vi "start.vi"(8 "error in (no error)":errorcluster, 11 "NetworkProEm in":refnum<class "Network_ProEm_WinX32.lvclass">) -> (0 "error out":errorcluster, 3 "NetworkProEM out":refnum<class "Network_ProEm_WinX32.lvclass">)   [LabVIEW 2009, in "Hardware.lvlib" / "HWControllers.lvlib" / "Network_ProEm_WinX32.lvclass"]
uses:
  Network_ProEm_WinX32.lvclass
  Channels/Camera/Camera/Camera.lvclass
  NetworkCamera.lvclass
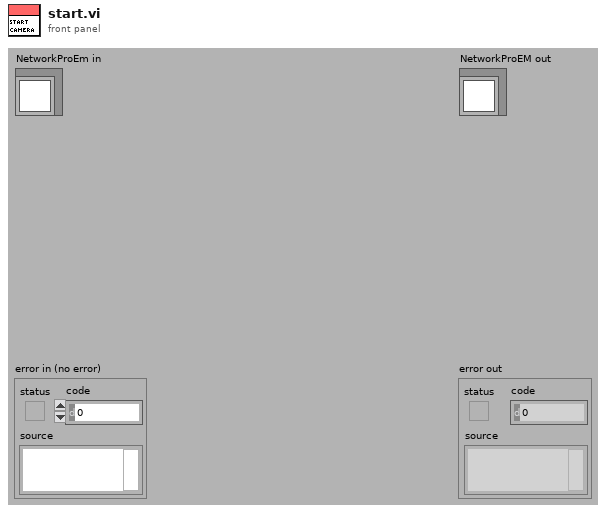
[diagram p1: front panel]
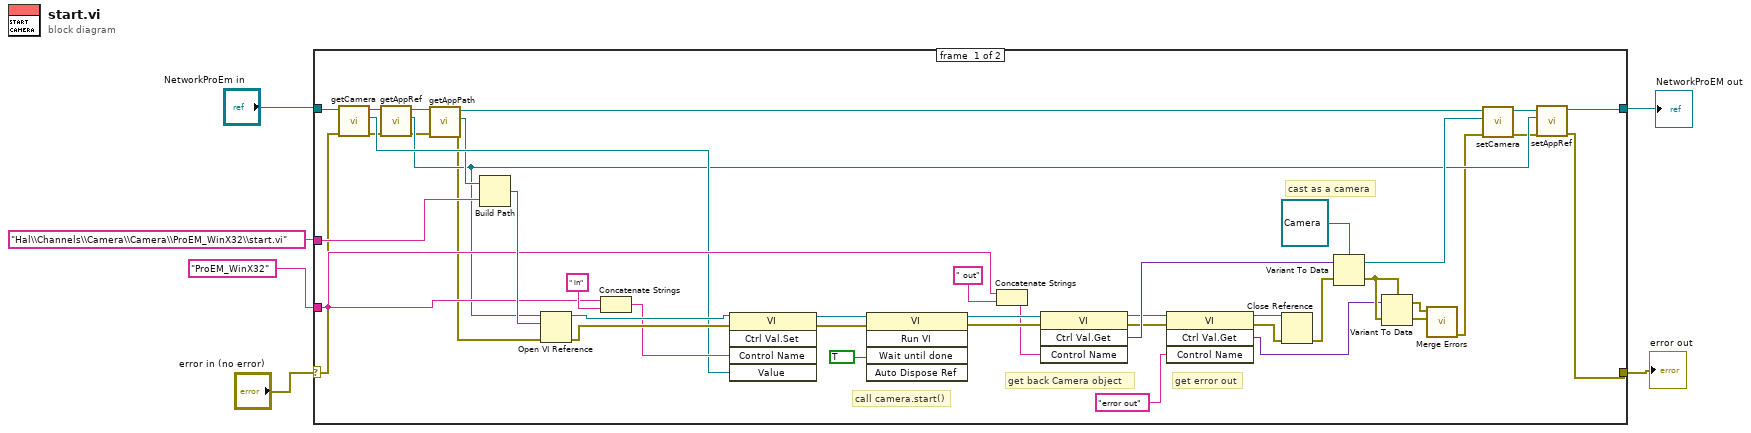
[diagram p0: block diagram]
diagram:
  n1 = case shown="No Error" "error in (no error)" {
    selector: "error in (no error)" -> [w8 w51]
    tunnel: [w21 w51] -> w2
    tunnel: [w26 w50] -> w1
    tunnel: "NetworkProEm in" -> [w31 w50]
    tunnel: "Hal\\Channels\\Camera\\Camera\\ProEM_WinX32\\start.vi" ("viPath") -> [w37 _]
    tunnel: "ProEM_WinX32" ("Control name") -> [w34 _]
    frame #0 {
      # "get error out"
      # "get back Camera object"
      # "call camera.start()"
      # "cast as a camera"
      n2 = call "getCamera.vi"("error in (no error)"=w8, "NetworkCamera in"=w31) -> ("error out"=w10:errorcluster, "Camera"=w28:refnum<class "Camera.lvclass">, "NetworkCamera out"=w30:refnum<class "Network_ProEm_WinX32.lvclass">)  [unwired: 7 in]
      n3 = call "getAppRef.vi"("error in (no error)"=w10, "NetworkCamera in"=w30) -> ("error out"=w9:errorcluster, "appRef"=w23:refnum<vi>, "NetworkCamera out"=w29:refnum<class "Network_ProEm_WinX32.lvclass">)  [unwired: 7 in]
      n4 = call "getAppPath.vi"("error in (no error)"=w9, "NetworkCamera in"=w29) -> ("error out"=w7:errorcluster, "appPath"=w27:path, "NetworkCamera out"=w25:refnum<class "Network_ProEm_WinX32.lvclass">)  [unwired: 7 in]
      n5 = Build Path(base path=w27, name or relative path=w37) -> (appended path=w49:path)
      n6 = Open VI Reference(application reference (local)=w23, vi path=w49, error in (no error)=w7) -> (vi reference=w39:refnum<vi>, error out=w38:errorcluster)  [unwired: 3 in]
      n7 = Concatenate Strings(w34, " in") -> (w35:string)
      n8 = invoke class="VI" method="Ctrl Val.Set"(reference=w39, error in=w38, "Control Name"=w35, "Value"=w28) -> (reference out=w48:refnum<vi>, error out=w47:errorcluster)  [unwired: 1 in, 3 out]
      n9 = invoke class="VI" method="Run VI"(reference=w48, error in=w47, "Wait until done"=TRUE) -> (reference out=w45:refnum<vi>, error out=w44:errorcluster)  [unwired: 2 in, 3 out]
      n10 = Concatenate Strings(w34, " out") -> (w32:string)
      n11 = invoke class="VI" method="Ctrl Val.Get"(reference=w45, error in=w44, "Control Name"=w32) -> (reference out=w41:refnum<vi>, error out=w18:errorcluster, "Get Control Value Variant"=w42:variant)  [unwired: 1 in, 1 out]
      n12 = invoke class="VI" method="Ctrl Val.Get"(reference=w41, error in=w18, "Control Name"="error out") -> (reference out=w19:refnum<vi>, error out=w17:errorcluster, "Get Control Value Variant"=w15:variant)  [unwired: 1 in, 1 out]
      n13 = Close Reference(reference=w19, error in (no error)=w17) -> (error out=w40:errorcluster)
      n14 = Variant To Data(error in=w40, Variant=w42, type=refnum<class "Camera.lvclass"> refnum ("Camera out")) -> (error out=w16:errorcluster, data=w24:refnum<class "Camera.lvclass">)
      n15 = Variant To Data(error in=w16, Variant=w15, type=w16) -> (error out=w14:errorcluster, data=w13:errorcluster)
      n16 = call <vilib>:"Merge Errors.vi"("error in 2 (no error)"=w14, "error in 1 (no error)"=w13) -> ("error out"=w12:errorcluster)  [unwired: 5 in]
      n17 = call "setCamera.vi"("error in (no error)"=w12, "Camera"=w24, "NetworkCamera in"=w25) -> ("error out"=w20:errorcluster, "NetworkCamera out"=w22:refnum<class "Network_ProEm_WinX32.lvclass">)  [unwired: 7 in]
      n18 = call "setAppRef.vi"("error in (no error)"=w20, "appRef"=w23, "NetworkCamera in"=w22) -> ("error out"=w21:errorcluster, "NetworkCamera out"=w26:refnum<class "Network_ProEm_WinX32.lvclass">)  [unwired: 7 in]
    }
    frame #1 {
    }
  }
  "error out" <- w2
  "NetworkProEM out" <- w1
